vi "Lin_Rohner_force_sensor_tachometer.vi"() -> ()   [LabVIEW 2019]
uses:
  <vilib>/Platform/TimedLoop/XDataNode/timing_clust.ctl
  <vilib>/Platform/TimedLoop/XDataNode/nitl_modes.ctl
  <vilib>/Platform/TimedLoop/XDataNode/wakeup.ctl
  <vilib>/Analysis/3filter.llb/Filter Passband Type.ctl
  <vilib>/DAQmx/write.llb/DAQmx Write (Analog DBL 1Chan 1Samp).vi
  <vilib>/DAQmx/read.llb/DAQmx Read (Analog 1D DBL NChan 1Samp).vi
  <vilib>/DAQmx/create/channels.llb/DAQmx Create Channel (AI-Voltage-Basic).vi
  <vilib>/DAQmx/create/channels.llb/DAQmx Create Channel (AO-Voltage-Basic).vi
  <vilib>/DAQmx/miscellaneous.llb/DAQmx Fill In Error Info.vi
  <vilib>/platform/TimedLoop/XDataNode/XDataNode.xnode
  <vilib>/Platform/TimedLoop/XDataNode/XDNodeRunTimeDep.lvlib
  <vilib>/ptbypt/NI_PtbyPt.lvlib
  <vilib>/Analysis/NI_AALBase.lvlib
panel:
  out "Filtered Paddle Angular Velocity(tachometer) [rad/s]":dbl
  out "Filtered Paddle Angular Velocity(tachometer) [rad/s]":dbl(graph)
  in  "low cutoff freq: paddle angular velocity(tachometer)":dbl=0.125 format="%0.3f"
  out "Raw Force [N]":dbl
  out "Raw Force [N]":dbl(graph)
  out "Filtered Paddle Angular Velocity(derivative) [rad/s]":dbl
  out "Filtered Paddle Angular Velocity(derivative) [rad/s]":dbl(graph)
  in  "low cutoff freq: angular velocity(derivative)":dbl=0.125 format="%0.3f"
  out "Raw Paddle Angular Velocity(tachometer) [rad/s]":dbl
  out "Raw Paddle Angular Velocity(tachometer) [rad/s]":dbl(graph)
  out "Raw Tachometer[V]":dbl
  out "Raw Tachometer[V]":dbl(graph)
  out "Filtered Force Sensor [V]":dbl
  out "Filtered Force Sensor [V]":dbl(graph)
  in  "low cutoff freq: force sensor)":dbl=0.125 format="%0.3f"
  out "Raw Force sensor [V]":dbl
  out "Raw Force sensor [V]":dbl(graph)
  out "Position [deg]":dbl(knob) scale=-32.5..32.5
  out "Filtered Position [deg]":dbl
  out "Filtered Postion Graph [deg]":dbl(graph)
  in  "stop":bool
  in  "low cutoff freq: position":dbl=0.125 format="%0.3f"
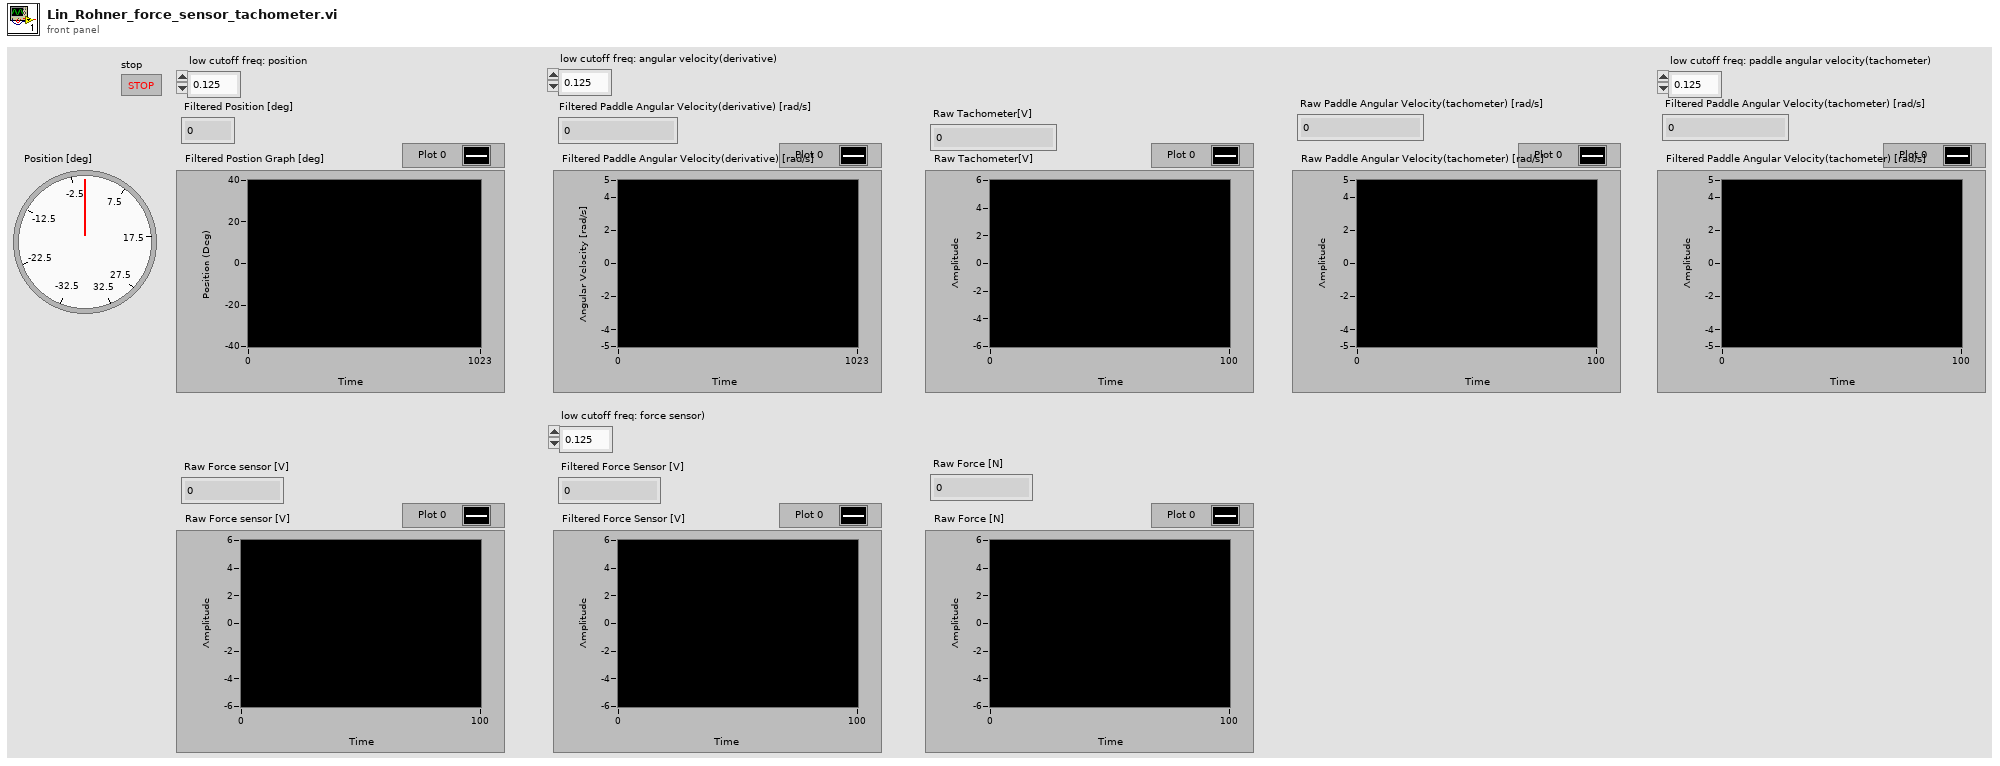
[diagram p1: front panel]
types:
  T1 = typedef "NI_AALBase.lvlib/Filter Passband Type.ctl" = enum32{"Lowpass", "Highpass", "Bandpass", "Bandstop"}
  T2 = typedef "XDNodeRunTimeDep.lvlib/timing_clust.ctl" = cluster{"Expected End [f-1]":u64, "Actual End [f-1]":u64, "Finished Late? [f-1]":bool, "Expected End [i-1]":u64, "Actual End [i-1]":u64, "Finished Late? [i-1]":bool, "Expected Start [i]":u64, "Actual Start [i]":u64, "Expected Start [f]":u64, "Actual Start [f]":u64, "Source Name":string, "Structure Name":string, "Period":i64, "Deadline":i64, "Offset":i64, "Start":i64, "Priority":i32, "Timeout":i32, "Mode":T3, "Wakeup Reason":T4, "Error":errorcluster, "Source Type":string, "Secondary Source Type":string, "Global End Time":u64, "Global Start Time":u64, "Frame Duration":u64, "Iteration Duration":u64, "Assigned CPU":i32, "I/O Scan Engine Mode":u32}
  T3 = typedef "XDNodeRunTimeDep.lvlib/nitl_modes.ctl" = enum32{"No Change", "Process missed periods, maintain original phase", "Discard missed periods, maintain original phase", "Process missed periods, ignore original phase", "Discard missed periods, ignore original phase"}
  T4 = typedef "XDNodeRunTimeDep.lvlib/wakeup.ctl" = enum32{"Normal", "Aborted", "Asynchronous wakeup", "Timing source error", "Timed loop error", "Timeout"}
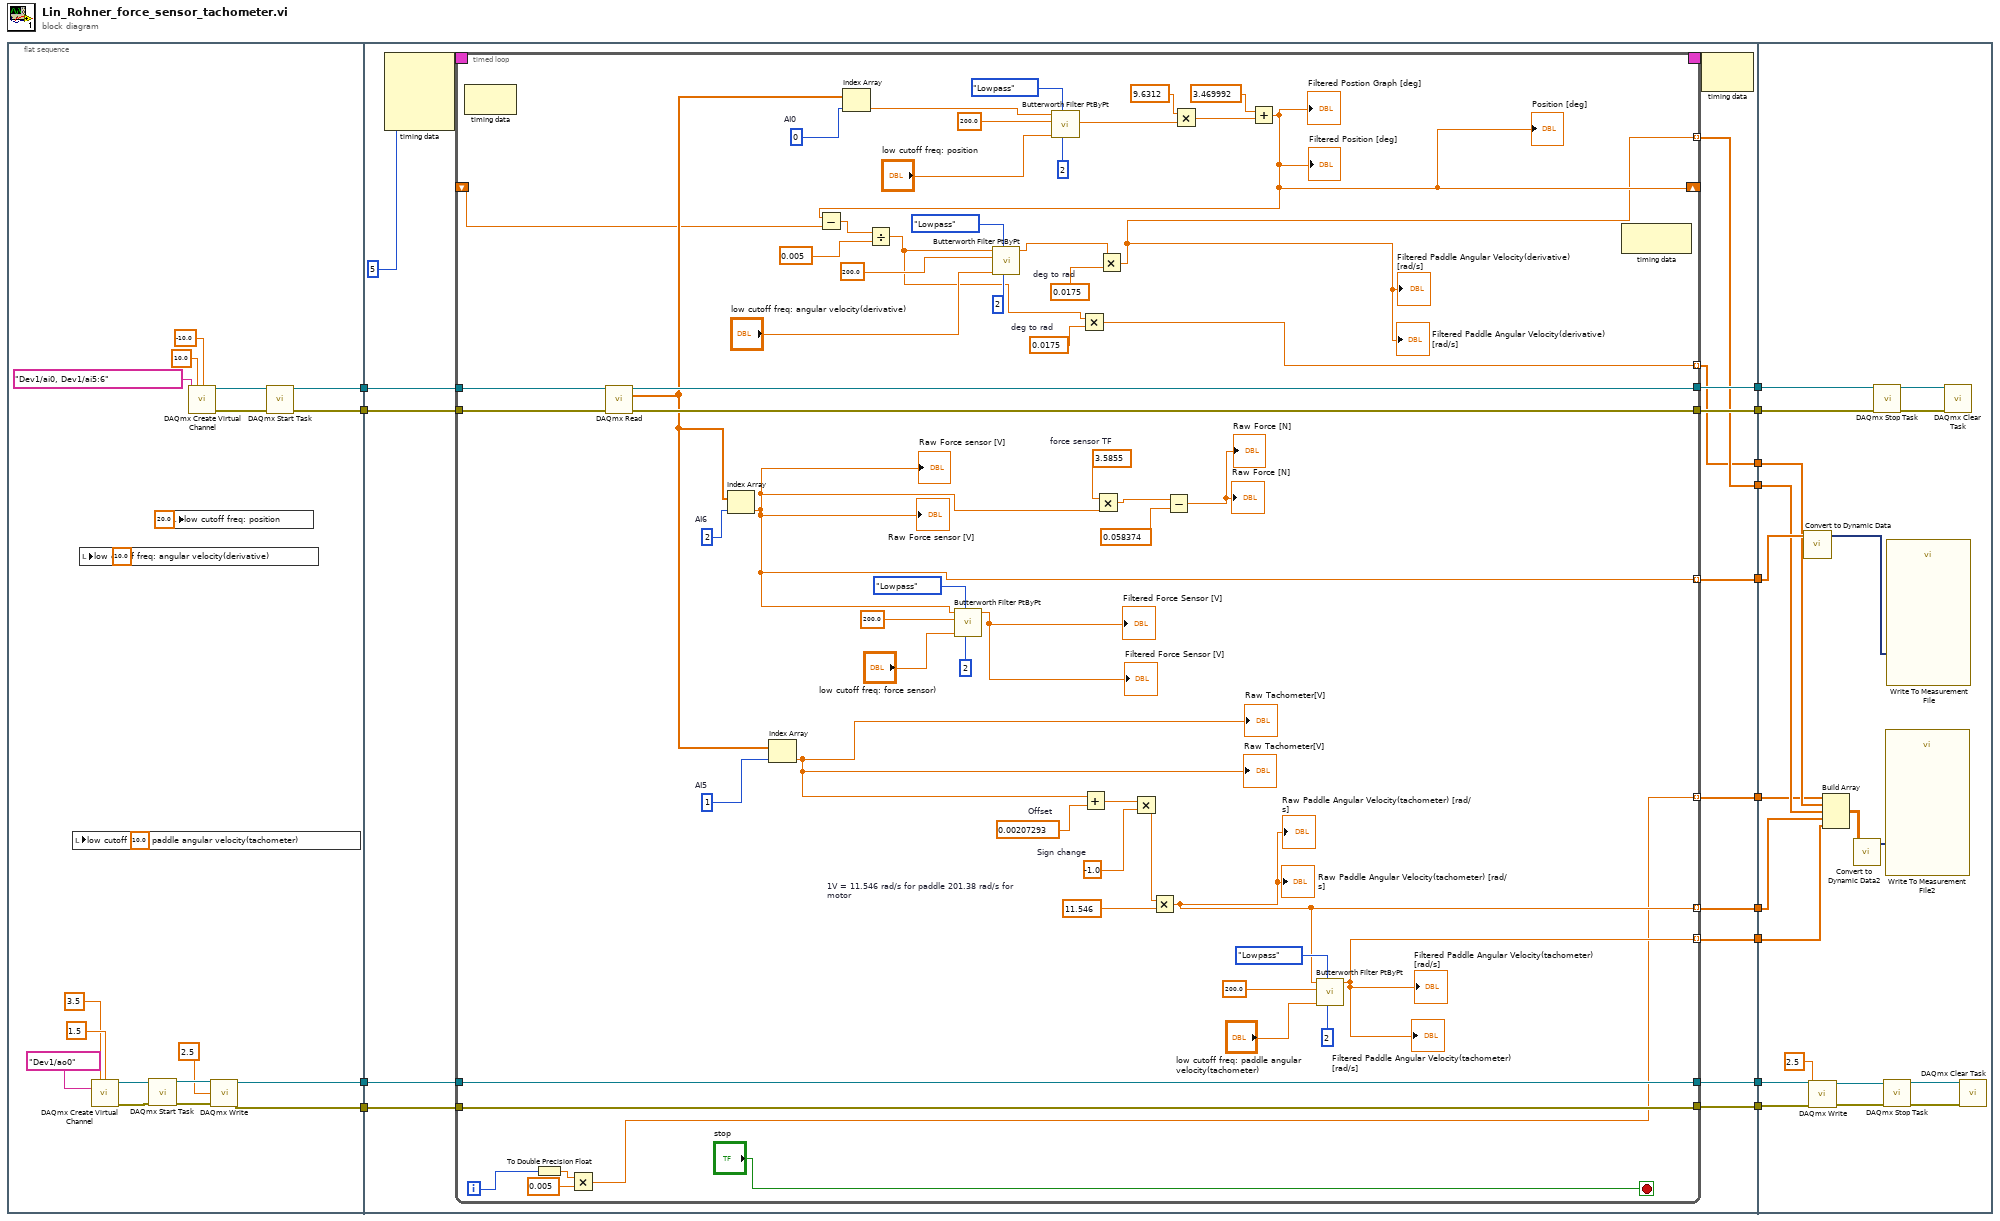
[diagram p0: block diagram]
diagram:
  n1 = flat-sequence {
    tunnel: [w31] -> w14
    tunnel: [w29] -> w12
    tunnel: [w19] -> w9
    tunnel: [w18] -> w8
    tunnel: w14 -> [w49]
    tunnel: [w48] -> w13
    tunnel: w12 -> [w47]
    tunnel: [w46] -> w11
    tunnel: [w44] -> w10
    tunnel: w9 -> [w43]
    tunnel: w8 -> [w42]
    tunnel: [w41] -> w7
    tunnel: [w40] -> w6
    tunnel: [w39] -> w5
    tunnel: [w38] -> w4
    tunnel: [w37] -> w3
    tunnel: [w36] -> w2
    tunnel: [w35] -> w1
    tunnel: w13 -> [w137]
    tunnel: w11 -> [w135]
    tunnel: w10 -> [w133]
    tunnel: w7 -> [w126]
    tunnel: w6 -> [w125]
    tunnel: w5 -> [w124]
    tunnel: w4 -> [w123]
    tunnel: w3 -> [w120]
    tunnel: w2 -> [w119]
    tunnel: w1 -> [w118]
    frame #0 {
      n2 = local write "low cutoff freq: paddle angular velocity(tachometer)"(10.0 ("filter Techometer 2")) -> ()
      n3 = local write "low cutoff freq: angular velocity(derivative)"(10.0 ("low cutoff freq: fl 3")) -> ()
      n4 = call-poly <vilib>:"DAQmx Create Virtual Channel.vi"("maximum value"=3.5, "minimum value"=1.5, "physical channels"=tag "Dev1/ao0") -> ("task out"=w27:refnum<k21>, "error out"=w25:errorcluster)  [unwired: 11 in]
      n5 = call <vilib>:"DAQmx Start Task.vi"("task/channels in"=w27, "error in"=w25) -> ("task out"=w26:refnum<k21>, "error out"=w24:errorcluster)  [unwired: 12 in]
      n6 = local write "low cutoff freq: position"(20.0 ("low cutoff freq: fl 2")) -> ()
      n7 = call-poly <vilib>:"DAQmx Create Virtual Channel.vi"("maximum value"=10.0, "minimum value"=-10.0, "physical channels"=tag "Dev1/ai0, Dev1/ai5:6") -> ("task out"=w30:refnum<k21>, "error out"=w32:errorcluster)  [unwired: 11 in]
      n8 = call-poly <vilib>:"DAQmx Write.vi"("task/channels in"=w26, "data"=2.5, "error in"=w24) -> ("task out"=w19:refnum<k21>, "error out"=w18:errorcluster)  [unwired: 10 in, 1 out]
      n9 = call <vilib>:"DAQmx Start Task.vi"("task/channels in"=w30, "error in"=w32) -> ("task out"=w29:refnum<k21>, "error out"=w31:errorcluster)  [unwired: 12 in]
    }
    frame #1 {
      n10 = node-c288(i64 5 ("Period")) -> (w51:T2)  [unwired: 3 in]
      n11 = timed-loop {
        timing: w51 -> [_]
        timing-out: [_] -> w50
        tunnel: w49 -> [w111]
        tunnel: [w110] -> w48
        tunnel: w47 -> [w106]
        tunnel: [w105] -> w46
        tunnel: [w70] -> w44 mode=indexing
        tunnel: w43 -> [w88]
        tunnel: w42 -> [w87]
        tunnel: [w88] -> w41
        tunnel: [w87] -> w40
        shift-right: [w80] -> _
        shift-left: _ -> [w79]
        tunnel: [w61] -> w39 mode=indexing
        tunnel: [w60] -> w38 mode=indexing
        tunnel: [w59] -> w37 mode=indexing
        tunnel: [w52] -> w36 mode=indexing
        tunnel: [w55] -> w35 mode=indexing
        i -> [w58]
        stop <- "stop" stop-if-true
        w53 = 0.0175  # deg to rad
        w69 = 3.5855  # force sensor TF
        w71 = 0.0175  # deg to rad
        w81 = 11.546  # 1V = 11.546 rad/s for paddle 201.38 rad/s for motor
        w83 = -1.0  # Sign change
        w85 = 0.00207293  # Offset
        w89 = 1  # AI5
        w96 = 2  # AI6
        w98 = 0  # AI0
        n12 = node-c288() -> ()  [unwired: 1 in, 1 out]
        n13 = To Double Precision Float(number=w58) -> (double precision float=w57:dbl)
        n14 = Multiply(x=w57, y=0.005) -> (x*y=w55:dbl)
        n15 = call-poly <vilib>:"DAQmx Read.vi"("task/channels in"=w106, "error in"=w111) -> ("task out"=w105:refnum<k21>, "data"=w90:dbl[], "error out"=w110:errorcluster)  [unwired: 11 in]
        n16 = Index Array(array=w90, index=w96) -> (element=w70:dbl)
        "Raw Force sensor [V]" <- w70
        "Raw Force sensor [V]" <- w70
        n17 = Index Array(array=w90, index=w89) -> (element=w86:dbl)
        "Raw Tachometer[V]" <- w86
        "Raw Tachometer[V]" <- w86
        n18 = Index Array(array=w90, index=w98) -> (element=w97:dbl)
        n19 = call <vilib>:"Butterworth Filter PtByPt.vi"("order"=2, "filter type"=Filter_Passband_Type."Lowpass", "low cutoff freq: fl"="low cutoff freq: force sensor)", "sampling freq: fs"=200.0, "x"=w70) -> ("Filtered x"=→"Filtered Force Sensor [V]" →"Filtered Force Sensor [V]":dbl)  [unwired: 4 in, 1 out]
        n20 = call <vilib>:"Butterworth Filter PtByPt.vi"("order"=2, "filter type"=Filter_Passband_Type."Lowpass", "low cutoff freq: fl"="low cutoff freq: position", "sampling freq: fs"=200.0, "x"=w97) -> ("Filtered x"=w99:dbl)  [unwired: 4 in, 1 out]
        n21 = Add(x=w86, y=w85) -> (x+y=w84:dbl)
        n22 = Multiply(x=w69, y=w70) -> (x*y=w68:dbl)
        n23 = Multiply(x=w84, y=w83) -> (x*y=w82:dbl)
        n24 = Multiply(x=w82, y=w81) -> (x*y=w61:dbl)
        "Raw Paddle Angular Velocity(tachometer) [rad/s]" <- w61
        "Raw Paddle Angular Velocity(tachometer) [rad/s]" <- w61
        n25 = Subtract(x=w68, y=0.058374) -> (x-y=→"Raw Force [N]" →"Raw Force [N]":dbl)
        n26 = Multiply(x=9.6312, y=w99) -> (x*y=w101:dbl)
        n27 = Add(x=3.469992, y=w101) -> (x+y=w80:dbl)
        "Filtered Postion Graph [deg]" <- w80
        "Filtered Position [deg]" <- w80
        "Position [deg]" <- w80
        n28 = Subtract(x=w80, y=w79) -> (x-y=w78:dbl)
        n29 = Divide(x=w78, y=0.005) -> (x/y=w54:dbl)
        n30 = call <vilib>:"Butterworth Filter PtByPt.vi"("order"=2, "filter type"=Filter_Passband_Type."Lowpass", "low cutoff freq: fl"="low cutoff freq: angular velocity(derivative)", "sampling freq: fs"=200.0, "x"=w54) -> ("Filtered x"=w72:dbl)  [unwired: 4 in, 1 out]
        n31 = Multiply(x=w54, y=w53) -> (x*y=w52:dbl)
        n32 = Multiply(x=w72, y=w71) -> (x*y=w59:dbl)
        "Filtered Paddle Angular Velocity(derivative) [rad/s]" <- w59
        "Filtered Paddle Angular Velocity(derivative) [rad/s]" <- w59
        n33 = call <vilib>:"Butterworth Filter PtByPt.vi"("order"=2, "filter type"=Filter_Passband_Type."Lowpass", "low cutoff freq: fl"="low cutoff freq: paddle angular velocity(tachometer)", "sampling freq: fs"=200.0, "x"=w61) -> ("Filtered x"=w60:dbl)  [unwired: 4 in, 1 out]
        "Filtered Paddle Angular Velocity(tachometer) [rad/s]" <- w60
        "Filtered Paddle Angular Velocity(tachometer) [rad/s]" <- w60
        n34 = node-c288() -> ()  [unwired: 1 in, 1 out]
      }
      n35 = node-c288(w50) -> ()  [unwired: 1 out]
    }
    frame #2 {
      n36 = call "Convert to Dynamic Data"("Array"=w133) -> ("Dynamic Data Type"=w132:dynamicdata)  [unwired: 3 in]
      n37 = call-poly <vilib>:"DAQmx Write.vi"("task/channels in"=w126, "data"=2.5, "error in"=w125) -> ("task out"=w131:refnum<k21>, "error out"=w128:errorcluster)  [unwired: 10 in, 1 out]
      n38 = Build Array(w118, w119, w120, w124, w123) -> (w122:dbl[][])
      n39 = call "Convert to Dynamic Data2"("2D Array"=w122) -> ("Dynamic Data Type"=w121:dynamicdata)  [unwired: 3 in]
      n40 = call <vilib>:"DAQmx Stop Task.vi"("task/channels in"=w135, "error in"=w137) -> ("task out"=w134:refnum<k21>, "error out"=w136:errorcluster)  [unwired: 12 in]
      n41 = call <vilib>:"DAQmx Stop Task.vi"("task/channels in"=w131, "error in"=w128) -> ("task out"=w130:refnum<k21>, "error out"=w129:errorcluster)  [unwired: 12 in]
      n42 = call "Write To Measurement File2"("Signals"=w121) -> ()  [unwired: 16 in, 3 out]
      n43 = call "Write To Measurement File"("Signals"=w132) -> ()  [unwired: 16 in, 3 out]
      n44 = call <vilib>:"DAQmx Clear Task.vi"("task in"=w134, "error in"=w136) -> ()  [unwired: 13 in, 1 out]
      n45 = call <vilib>:"DAQmx Clear Task.vi"("task in"=w130, "error in"=w129) -> ()  [unwired: 13 in, 1 out]
    }
  }
